vi "measuring loop time.vi"() -> ()   [LabVIEW 2018]
panel:
  out "Loop Iteration":i32
  in  "stop":bool
  out "loop time [ms]":u32
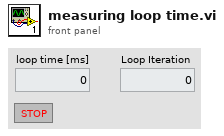
[diagram p1: front panel]
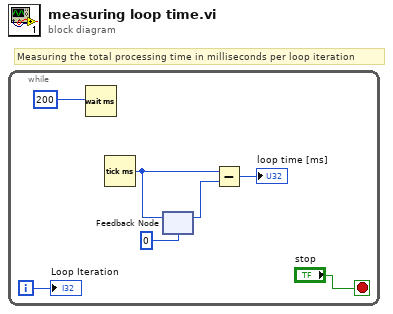
[diagram p0: block diagram]
diagram:
  # "Measuring the total processing time in milliseconds per loop iteration"
  n1 = while {
    i -> [w1]
    stop <- "stop" stop-if-true
    n2 = Wait (ms)(milliseconds to wait=200) -> ()  [unwired: 1 out]
    n3 = Tick Count (ms)() -> (millisecond timer value=w5:u32)
    n4 = feedback-in #1(w5) -> ()
    n5 = feedback #1(0) -> (w6:u32)
    n6 = Subtract(x=w5, y=w6) -> (x-y=→"loop time [ms]":u32)
    "Loop Iteration" <- w1
  }
